vi "Load_Program.vi"(2 "error in (no error)":errorcluster, 3 "FLASH":bool, 4 "Queue in":refnum<queue>) -> (0 "error out":errorcluster, 1 "Queue out":refnum<queue>)   [LabVIEW 2017]
panel:
  out "Array 3":bool[](array[boolean])
  out "Array 2":bool[](array[boolean])
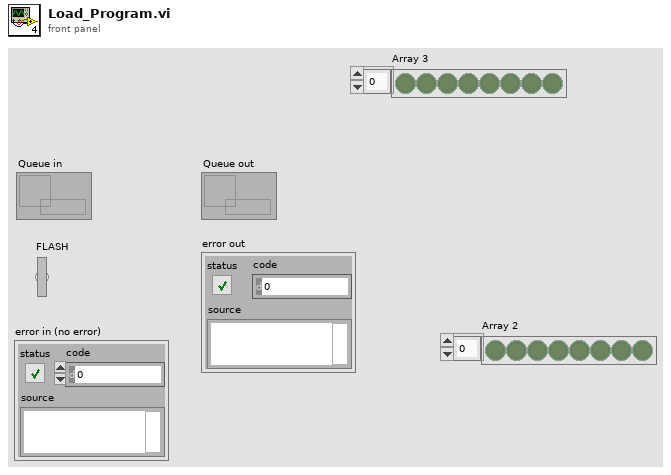
[diagram p1: front panel]
types:
  T1 = enum16{"Write Enable", "Page Program", "Write Disable", "Read Status", "Read Memory", "Program FPGA"}
  T2 = enum16{"Set Data", "Set Write", "Unset Write", "Unset Data"}
  T3 = enum16{"Write Enable", "Page Program", "Write Disable", "Read Status", "Read Memory"}
  T4 = enum16{"Write Enable", "Page Program", "Write Disable", "Read Status"}
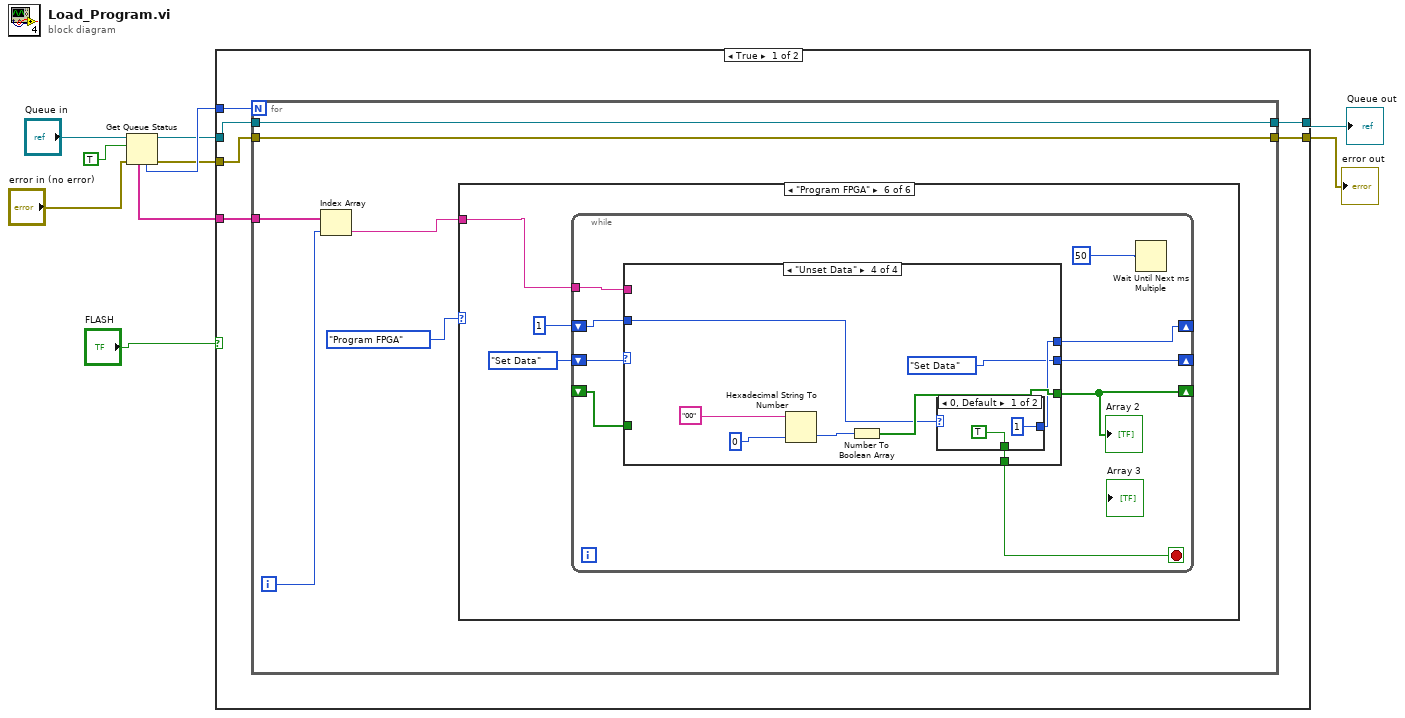
[diagram p0: block diagram]
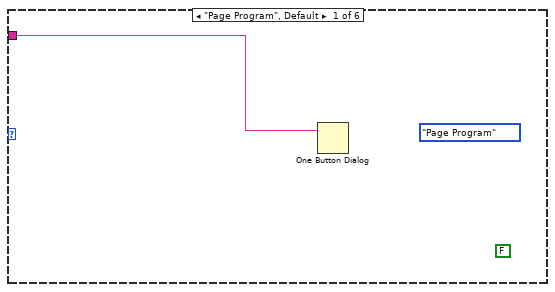
[diagram p2: hidden frame]
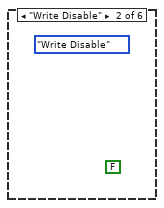
[diagram p3: hidden frame]
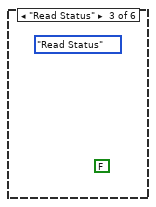
[diagram p4: hidden frame]
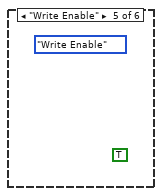
[diagram p6: hidden frame]
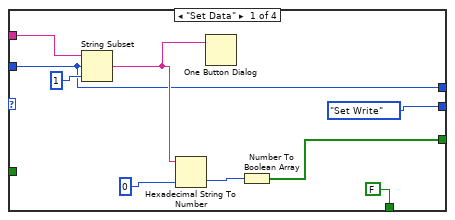
[diagram p7: hidden frame]
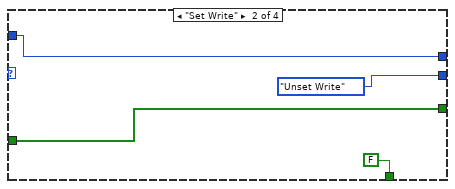
[diagram p8: hidden frame]
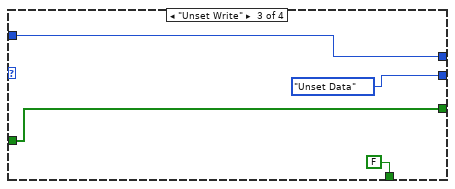
[diagram p9: hidden frame]
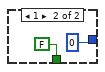
[diagram p10: hidden frame]
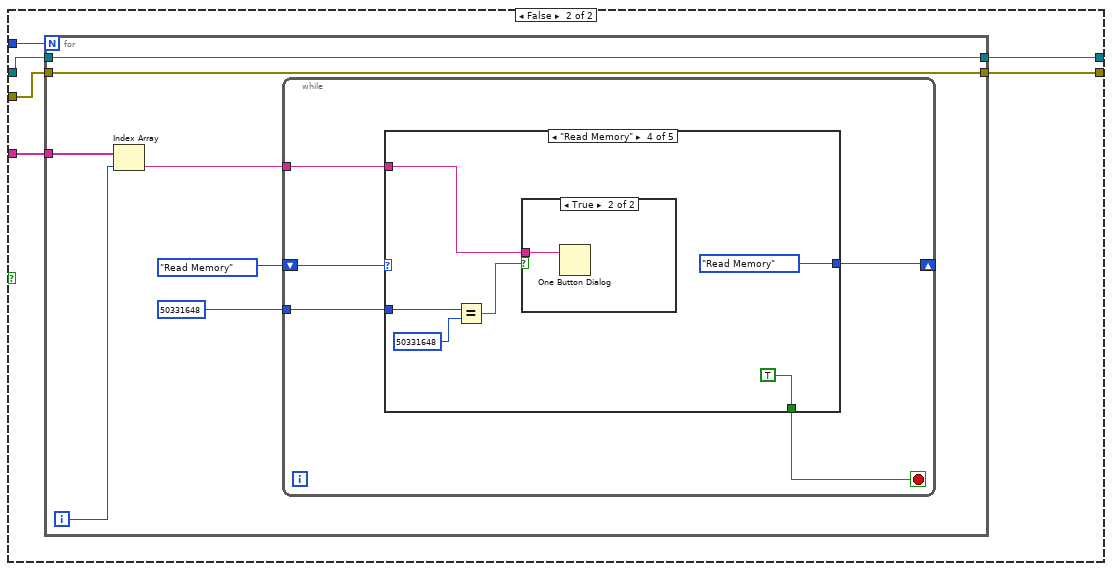
[diagram p11: hidden frame]
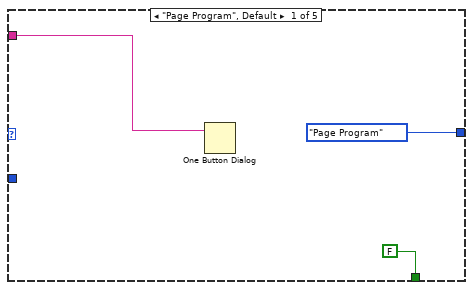
[diagram p12: hidden frame]
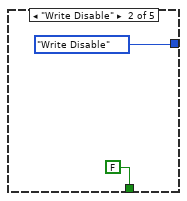
[diagram p13: hidden frame]
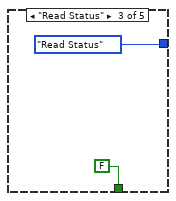
[diagram p14: hidden frame]
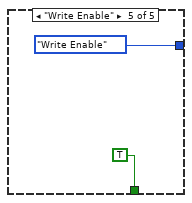
[diagram p16: hidden frame]
diagram:
  n1 = Get Queue Status(queue="Queue in", return elements? (F)=TRUE, error in (no error)="error in (no error)") -> (queue out=w5:refnum<queue>, error out=w3:errorcluster, # elements in queue=w9:i32, elements=w6:string[])  [unwired: 4 out]
  n2 = case shown="True" "FLASH" {
    tunnel: w9 -> [w16 w70]
    tunnel: w6 -> [w15 w69]
    tunnel: w5 -> [w14 w68]
    tunnel: [w13 w67] -> w4
    tunnel: w3 -> [w12 w66]
    tunnel: [w11 w65] -> w1
    frame True {
      n3 = for {
        N: w16 -> [_]
        tunnel: w15 -> [w22]
        tunnel: w14 -> [w20]
        tunnel: [w20] -> w13
        tunnel: w12 -> [w19]
        tunnel: [w19] -> w11
        i -> [w21]
        n4 = Index Array(array=w22, index=w21) -> (element=w17:string)
        n5 = case shown="\"Program FPGA\"" T1."Program FPGA" {
          tunnel: w17 -> [w23 _ _ _ _ w26]
          frame "Page Program", Default {
            (unwired) FALSE
            (unwired) T4."Page Program"
            n6 = One Button Dialog(message=w23) -> ()  [unwired: 1 in, 1 out]
          }
          frame "Write Disable" {
            (unwired) FALSE
            (unwired) T4."Write Disable"
          }
          frame "Read Status" {
            (unwired) FALSE
            (unwired) T4."Read Status"
          }
          frame "Read Memory" {
          }
          frame "Write Enable" {
            (unwired) TRUE
            (unwired) T4."Write Enable"
          }
          frame "Program FPGA" {
            n7 = while {
              tunnel: w26 -> [w35]
              shift-right: [w33] -> _
              shift-left: _ -> [w34]
              shift-right: [w29] -> _
              shift-left: 1 -> [w30]
              shift-right: [w27] -> _
              shift-left: T2."Set Data" -> [w28]
              stop <- w32 stop-if-true
              n8 = case shown="\"Unset Data\"" w28 {
                tunnel: w35 -> [w40 _ _ _]
                tunnel: [w43 w48 w52 w57] -> w33
                tunnel: w34 -> [_ w48 w52 _]
                tunnel: [FALSE FALSE FALSE w56] -> w32
                tunnel: w30 -> [w37 w46 w50 w55]
                tunnel: [w37 w46 w50 w54] -> w29
                tunnel: [T2."Set Write" T2."Unset Write" T2."Unset Data" T2."Set Data"] -> w27
                frame "Set Data" {
                  n9 = String Subset(string=w40, offset (0)=w37, length (rest)=1) -> (substring=w38:string)
                  n10 = Hexadecimal String To Number(string=w38, default (0uL)=u8 0) -> (number=w44:u8)  [unwired: 1 in, 1 out]
                  n11 = One Button Dialog(message=w38) -> ()  [unwired: 1 in, 1 out]
                  n12 = Number To Boolean Array(number=w44) -> (Boolean array=w43:bool[])
                }
                frame "Set Write" {
                }
                frame "Unset Write" {
                }
                frame "Unset Data" {
                  n13 = Hexadecimal String To Number(string="00", default (0uL)=u8 0) -> (number=w60:u8)  [unwired: 1 in, 1 out]
                  n14 = Number To Boolean Array(number=w60) -> (Boolean array=w57:bool[])
                  n15 = case shown="0, Default" w55 {
                    tunnel: [TRUE FALSE] -> w56
                    tunnel: [1 0] -> w54
                    frame 0, Default {
                    }
                    frame 1 {
                    }
                  }
                }
              }
              "Array 2" <- w33
              n16 = Wait Until Next ms Multiple(millisecond multiple=50) -> ()  [unwired: 1 out]
            }
          }
        }
      }
    }
    frame False {
      n17 = for {
        N: w70 -> [_]
        tunnel: w69 -> [w77]
        tunnel: w68 -> [w73]
        tunnel: [w73] -> w67
        tunnel: w66 -> [w72]
        tunnel: [w72] -> w65
        i -> [w76]
        n18 = Index Array(array=w77, index=w76) -> (element=w74:string)
        n19 = while {
          shift-right: [w81] -> _
          shift-left: T3."Read Memory" -> [w82]
          tunnel: w74 -> [w79]
          tunnel: 50331648 -> [w78]
          stop <- w80 stop-if-true
          n20 = case shown="\"Read Memory\"" w82 {
            tunnel: [T4."Page Program" T4."Write Disable" T4."Read Status" T3."Read Memory" T4."Write Enable"] -> w81
            tunnel: [FALSE FALSE FALSE TRUE TRUE] -> w80
            tunnel: w79 -> [w83 _ _ w94 _]
            tunnel: w78 -> [_ _ _ w91 _]
            frame "Page Program", Default {
              n21 = One Button Dialog(message=w83) -> ()  [unwired: 1 in, 1 out]
            }
            frame "Write Disable" {
            }
            frame "Read Status" {
            }
            frame "Read Memory" {
              n22 = Equal?(x=w91, y=50331648) -> (x = y?=w90:bool)
              n23 = case shown="True" w90 {
                tunnel: w94 -> [_ w96]
                frame False {
                }
                frame True {
                  n24 = One Button Dialog(message=w96) -> ()  [unwired: 1 in, 1 out]
                }
              }
            }
            frame "Write Enable" {
            }
          }
        }
      }
    }
  }
  "Queue out" <- w4
  "error out" <- w1
